vi "data insert core.vi"(8 "error in (no error)":errorcluster, 9 "column information":T1[](array[typedef]), 10 "data":variant[](array[variant]), 11 "table":string) -> (0 "error out":errorcluster)   [LabVIEW 2016, in "采配水.lvlib"]
uses:
  <vilib>/addons/database/Auxilliary.llb/DB Tools Column Info.ctl
  <vilib>/addons/database/Auxilliary.llb/DB Tools DataTypes.ctl
  <vilib>/Utility/sysdir.llb/System Directory Type.ctl
  <vilib>/addons/database/Auxilliary.llb/DB Tools Transaction.ctl
  <vilib>/addons/database/Auxilliary.llb/DB Tools Isolation Level.ctl
  <vilib>/addons/database/Auxilliary.llb/DB Tools Parameter Info.ctl
  <vilib>/addons/database/Auxilliary.llb/DB Tools Parameter Dir.ctl
  <vilib>/addons/database/Connection.llb/DB Tools Open Connec (String).vi
  <vilib>/addons/database/Connection.llb/Conn Transaction.vi
  <vilib>/addons/database/Connection.llb/Conn Execute.vi
  <vilib>/addons/database/Recordset.llb/Rec Destroy - Connection.vi
  <vilib>/addons/database/Command.llb/Cmd Set Parameter Value (C).vi
  <vilib>/addons/database/Auxilliary.llb/DB Tools Format Datetime String (Time Stamp).vi
  <vilib>/addons/database/Command.llb/Cmd Execute.vi
  <vilib>/addons/database/Recordset.llb/Rec Destroy - Command.vi
  <vilib>/addons/database/Command.llb/Cmd Delete.vi
  <vilib>/addons/database/NI_Database_API.lvlib
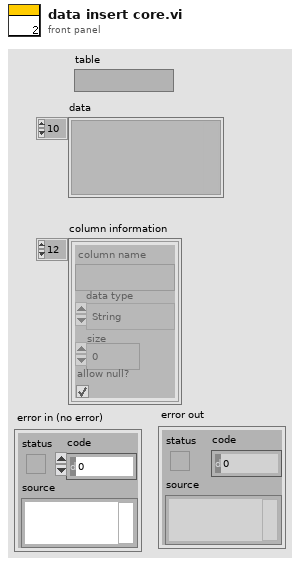
[diagram p1: front panel]
types:
  T1 = typedef "NI_Database_API.lvlib/DB Tools Column Info.ctl" = cluster{"column name":string, "data type":T2, "size":i32, "allow null?":bool}
  T2 = typedef "NI_Database_API.lvlib/DB Tools DataTypes.ctl" = enum16{"String", "Long (I32)", "Single (SGL)", "Double (DBL)", "Date/Time", "Binary"}
  T3 = typedef "NI_Database_API.lvlib/DB Tools Isolation Level.ctl" = enum16{"chaos", "read uncommitted", "read committed", "repeatable read", "serializable"}
  T4 = typedef "NI_Database_API.lvlib/DB Tools Transaction.ctl" = enum16{"begin", "commit", "rollback"}
  T5 = typedef "System Directory Type.ctl" = i32
  T6 = typedef "NI_Database_API.lvlib/Conn ObjectReference.ctl" = refnum<k1>
  T7 = typedef "NI_Database_API.lvlib/DB Tools Parameter Info.ctl" = cluster{"parameter name":string, "type":T2, "direction":T8, "value":variant}
  T8 = typedef "NI_Database_API.lvlib/DB Tools Parameter Dir.ctl" = enum32{"Input", "Output", "Input/Output", "Return Value"}
  T9 = typedef "NI_Database_API.lvlib/Rec ObjectReference.ctl" = refnum<k1>
  T10 = typedef "NI_Database_API.lvlib/Cmd ObjectReference.ctl" = refnum<k1>
  T11 = typedef "NI_Database_API.lvlib/Cmd-Rec Object Reference.ctl" = refnum<k1>
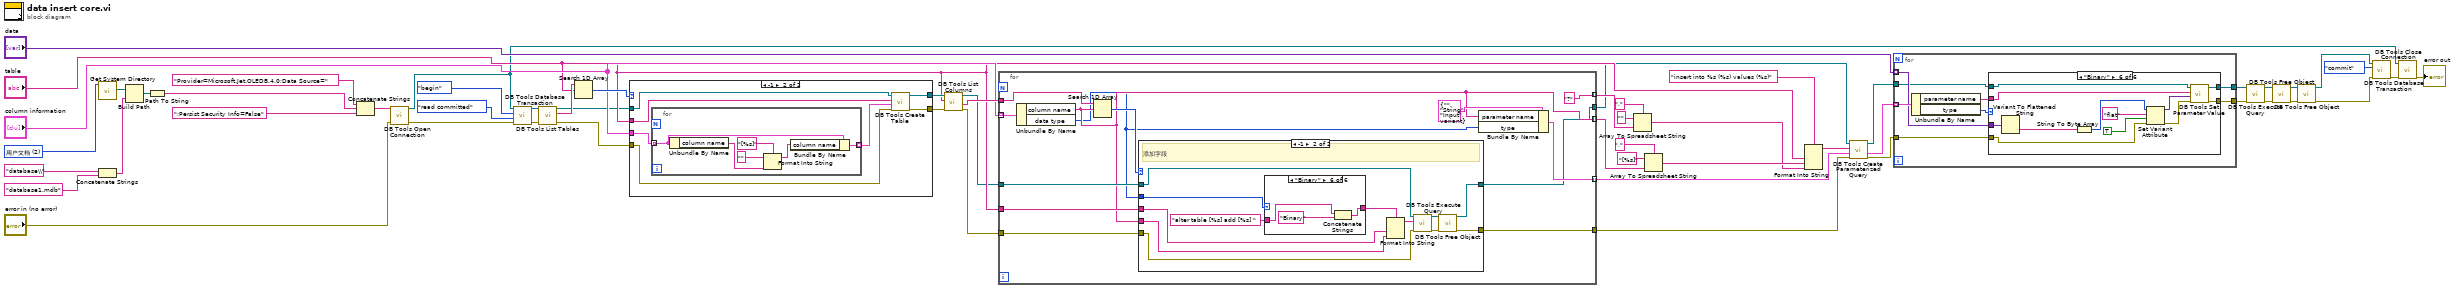
[diagram p0: block diagram]
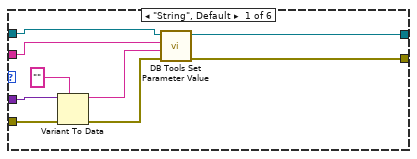
[diagram p2: hidden frame]
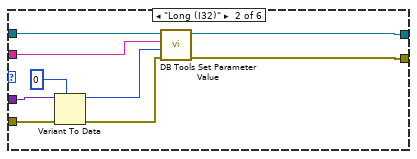
[diagram p3: hidden frame]
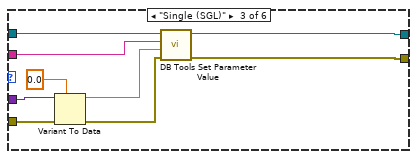
[diagram p4: hidden frame]
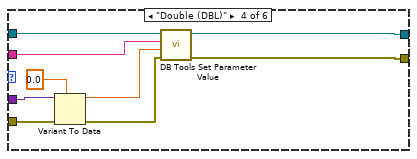
[diagram p5: hidden frame]
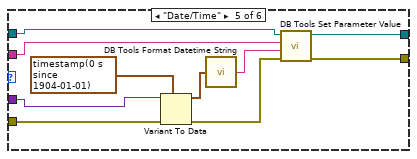
[diagram p6: hidden frame]
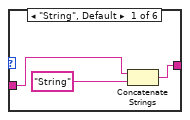
[diagram p8: hidden frame]
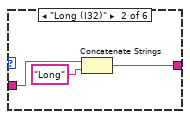
[diagram p9: hidden frame]
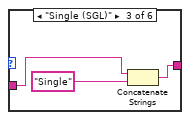
[diagram p10: hidden frame]
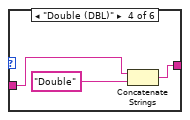
[diagram p11: hidden frame]
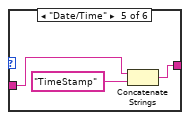
[diagram p12: hidden frame]
diagram:
  w56 = T5 2 items=["用户目录"=0, "用户桌面"=1, "用户文档"=2, "用户应用程序数据"=3, "用户设置"=4, "用户临时目录"=5, "公共文档"=6, "公共应用程序数据"=7, "公共设置"=8, "公共缓存"=13, "系统核心库"=9, "系统安装库"=10, "应用程序文件"=11, "启动盘根目录"=12] ("system directory type")
  n1 = call <vilib>:"Get System Directory.vi"("system directory type"=w56) -> ("system directory"=w54:path)  [unwired: 10 in]
  n2 = Concatenate Strings("database\\" ("condition"), "database1.mdb" ("database")) -> (w48:string)
  n3 = Build Path(base path=w54, name or relative path=w48) -> (appended path=w53:path)
  n4 = Path To String(path=w53) -> (string=w52:string)
  n5 = Concatenate Strings("Provider=Microsoft.Jet.OLEDB.4.0;Data Source=" ("condition"), w52, ";Persist Security Info=False" ("condition")) -> (w50:string)
  n6 = call-poly <vilib>:"DB Tools Open Connection.vi"("error in (no error)"="error in (no error)", "connection information"=w50) -> ("error out"=w9:errorcluster, "connection reference"=w1:T6)  [unwired: 6 in]
  n7 = call-poly <vilib>:"DB Tools Database Transaction.vi"("error in (no error)"=w9, "isolation level (chaos)"=DB_Tools_Isolation_Level."read committed", "operation (begin)"=DB_Tools_Transaction."begin", "connection reference"=w1) -> ("error out"=w8:errorcluster, "connection reference out"=w10:T6)  [unwired: 2 in]
  n8 = call <vilib>:"DB Tools List Tables.vi"("error in (no error)"=w8, "connection reference"=w10) -> ("error out"=w39:errorcluster, "tables"=w41:string[], "connection reference out"=w4:T6)  [unwired: 3 in]
  n9 = Search 1D Array(1D array=w41, element="table") -> (index of element=w40:i32)  [unwired: 1 in]
  n10 = case shown="-1" w40 {
    tunnel: w4 -> [w58 w65]
    tunnel: w39 -> [w57 w64]
    tunnel: "table" -> [_ w63]
    tunnel: "column information" -> [_ w60]
    tunnel: [w58 w62] -> w35
    tunnel: [w57 w61] -> w34
    frame 0, Default {
    }
    frame -1 {
      n11 = for {
        tunnel: w60 -> [w67] mode=indexing
        tunnel: [w66] -> w59 mode=indexing
        n12 = Unbundle By Name(w67) -> ("column name"=w71:string)
        n13 = Format Into String(format string="[%s]" ("格式字符串"), initial string="" ("初始字符串"), w71) -> (resulting string=w68:string)  [unwired: 1 in, 1 out]
        n14 = Bundle By Name(cluster=w67, "column name"=w68) -> (w66:T1)
      }
      n15 = call <vilib>:"DB Tools Create Table.vi"("error in (no error)"=w64, "column information"=w59, "table"=w63, "connection reference"=w65) -> ("error out"=w61:errorcluster, "connection reference out"=w62:T6)  [unwired: 4 in]
    }
  }
  n16 = call <vilib>:"DB Tools List Columns.vi"("error in (no error)"=w34, "table"="table", "connection reference"=w35) -> ("error out"=w37:errorcluster, "columns"=w38:string[], "connection reference out"=w6:T6)  [unwired: 1 in, 1 out]
  n17 = for {
    tunnel: w6 -> [w82]
    tunnel: w38 -> [w84]
    tunnel: w37 -> [w81]
    tunnel: [w80] -> w33
    tunnel: "table" -> [w79]
    tunnel: "column information" -> [w78] mode=indexing
    tunnel: [w76] -> w32 mode=indexing
    tunnel: [w75] -> w25 mode=indexing
    tunnel: ["?"] -> w23 mode=indexing
    tunnel: [w72] -> w3
    n18 = Unbundle By Name(w78) -> ("column name"=w75:string, "data type"=w73:T2)
    n19 = Search 1D Array(1D array=w84, element=w75) -> (index of element=w83:i32)  [unwired: 1 in]
    n20 = case shown="-1" w83 {
      tunnel: [w86 w95] -> w80
      tunnel: w82 -> [w85 w94]
      tunnel: w75 -> [_ w93]
      tunnel: w81 -> [w86 w92]
      tunnel: w79 -> [_ w91]
      tunnel: w73 -> [_ w89]
      tunnel: [w85 w87] -> w72
      frame 0, Default {
      }
      frame -1 {
        # "添加字段"
        n21 = case shown="\"Binary\"" w89 {
          tunnel: "alter table [%s] add [%s] " -> [w101 w104 w107 w110 w113 w116]
          tunnel: [w100 w103 w106 w109 w112 w115] -> w88
          frame "String", Default {
            n22 = Concatenate Strings(w101, "String" ("字符串")) -> (w100:string)
          }
          frame "Long (I32)" {
            n23 = Concatenate Strings(w104, "Long" ("字符串")) -> (w103:string)
          }
          frame "Single (SGL)" {
            n24 = Concatenate Strings(w107, "Single" ("字符串")) -> (w106:string)
          }
          frame "Double (DBL)" {
            n25 = Concatenate Strings(w110, "Double" ("字符串")) -> (w109:string)
          }
          frame "Date/Time" {
            n26 = Concatenate Strings(w113, "TimeStamp" ("字符串")) -> (w112:string)
          }
          frame "Binary" {
            n27 = Concatenate Strings(w116, "Binary" ("字符串")) -> (w115:string)
          }
        }
        n28 = Format Into String(format string=w88, w91, w93) -> (resulting string=w96:string)  [unwired: 2 in, 1 out]
        n29 = call-poly <vilib>:"DB Tools Execute Query.vi"("error in (no error)"=w92, "SQL query"=w96, "connection reference"=w94) -> ("error out"=w97:errorcluster, "recordset reference"=w98:T9)  [unwired: 5 in]
        n30 = call-poly <vilib>:"DB Tools Free Object.vi"("error in (no error)"=w97, "recordset reference"=w98) -> ("error out"=w95:errorcluster, "connection reference"=w87:T6)  [unwired: 8 in]
      }
    }
    n31 = Bundle By Name(cluster=T7 {"parameter name"="", "type"=enum."String", "direction"=enum."Input", "value"=variant} ("parameter information"), "parameter name"=w75, "type"=w73) -> (w76:T7)
  }
  n32 = Array To Spreadsheet String(delimiter (Tab)="," ("分隔符(Tab)"), array=w23, 3:"" ("格式字符串")) -> (spreadsheet string=w22:string)
  n33 = Array To Spreadsheet String(delimiter (Tab)="," ("分隔符(Tab)"), array=w25, 3:"[%s]" ("格式字符串")) -> (spreadsheet string=w24:string)
  n34 = Format Into String(format string="insert into %s (%s) values (%s)" ("格式字符串"), "table", w24, w22) -> (resulting string=w21:string)  [unwired: 2 in, 1 out]
  n35 = call <vilib>:"DB Tools Create Parameterized Query.vi"("error in (no error)"=w33, "parameters"=w32, "SQL query"=w21, "connection reference"=w3) -> ("error out"=w20:errorcluster, "parameters out"=w19:T7[], "command reference"=w5:T10)  [unwired: 3 in]
  n36 = for {
    tunnel: w5 -> [w121]
    tunnel: w20 -> [w119]
    tunnel: w19 -> [w124] mode=indexing
    tunnel: "data" -> [w122] mode=indexing
    tunnel: [w118] -> w2
    tunnel: [w117] -> w18
    n37 = Unbundle By Name(w124) -> ("parameter name"=w120:string, "type"=w123:T2)
    n38 = case shown="\"Binary\"" w123 {
      tunnel: w122 -> [w128 w136 w143 w153 w170 w174]
      tunnel: w121 -> [w131 w140 w147 w157 w168 w182]
      tunnel: w120 -> [w130 w139 w146 w152 w167 w181]
      tunnel: w119 -> [w125 w134 w144 w154 w165 w173]
      tunnel: [w127 w138 w148 w156 w164 w180] -> w118
      tunnel: [w126 w137 w145 w155 w163 w179] -> w117
      frame "String", Default {
        n39 = Variant To Data(error in=w125, type="", Variant=w128) -> (data=w129:string, error out=w133:errorcluster)
        n40 = call-poly <vilib>:"DB Tools Set Parameter Value.vi"("error in (no error)"=w133, "value"=w129, "parameter index"=w130, "command reference"=w131) -> ("error out"=w126:errorcluster, "command reference out"=w127:T10)  [unwired: 4 in]
      }
      frame "Long (I32)" {
        n41 = Variant To Data(error in=w134, type=0, Variant=w136) -> (data=w141:i32, error out=w142:errorcluster)
        n42 = call-poly <vilib>:"DB Tools Set Parameter Value.vi"("error in (no error)"=w142, "value"=w141, "parameter index"=w139, "command reference"=w140) -> ("error out"=w137:errorcluster, "command reference out"=w138:T10)  [unwired: 4 in]
      }
      frame "Single (SGL)" {
        n43 = Variant To Data(error in=w144, type=sgl 0.0, Variant=w143) -> (data=w150:sgl, error out=w151:errorcluster)
        n44 = call-poly <vilib>:"DB Tools Set Parameter Value.vi"("error in (no error)"=w151, "value"=w150, "parameter index"=w146, "command reference"=w147) -> ("error out"=w145:errorcluster, "command reference out"=w148:T10)  [unwired: 4 in]
      }
      frame "Double (DBL)" {
        n45 = Variant To Data(error in=w154, type=0.0, Variant=w153) -> (data=w159:dbl, error out=w160:errorcluster)
        n46 = call-poly <vilib>:"DB Tools Set Parameter Value.vi"("error in (no error)"=w160, "value"=w159, "parameter index"=w152, "command reference"=w157) -> ("error out"=w155:errorcluster, "command reference out"=w156:T10)  [unwired: 4 in]
      }
      frame "Date/Time" {
        n47 = Variant To Data(error in=w165, type=timestamp(0 s since 1904-01-01) ("时间标识"), Variant=w170) -> (data=w162:timestamp, error out=w166:errorcluster)
        n48 = call-poly <vilib>:"DB Tools Format Datetime String.vi"("time stamp"=w162) -> ("date/time string"=w161:string)
        n49 = call-poly <vilib>:"DB Tools Set Parameter Value.vi"("error in (no error)"=w166, "value"=w161, "parameter index"=w167, "command reference"=w168) -> ("error out"=w163:errorcluster, "command reference out"=w164:T10)  [unwired: 4 in]
      }
      frame "Binary" {
        n50 = Variant To Flattened String(Variant=w174) -> (data string=w175:string)  [unwired: 1 out]
        n51 = String To Byte Array(string=w175) -> (unsigned byte array=w178:u8[])
        n52 = Set Variant Attribute(Variant=w178, name="flat", value=TRUE, error in=w173) -> (Variant out=w171:variant, error out=w172:errorcluster)  [unwired: 1 out]
        n53 = call-poly <vilib>:"DB Tools Set Parameter Value.vi"("error in (no error)"=w172, "value"=w171, "parameter index"=w181, "command reference"=w182) -> ("error out"=w179:errorcluster, "command reference out"=w180:T10)  [unwired: 4 in]
      }
    }
  }
  n54 = call-poly <vilib>:"DB Tools Execute Query.vi"("error in (no error)"=w18, "command reference"=w2) -> ("error out"=w16:errorcluster, "command-recordset reference"=w17:T11)  [unwired: 6 in]
  n55 = call-poly <vilib>:"DB Tools Free Object.vi"("error in (no error)"=w16, "command-recordset reference"=w17) -> ("error out"=w14:errorcluster, "command reference"=w15:T10)  [unwired: 8 in]
  n56 = call-poly <vilib>:"DB Tools Free Object.vi"("error in (no error)"=w14, "command reference"=w15) -> ("error out"=w11:errorcluster, "connection reference"=w12:T6)  [unwired: 8 in]
  n57 = call-poly <vilib>:"DB Tools Database Transaction.vi"("error in (no error)"=w11, "operation (begin)"=DB_Tools_Transaction."commit", "connection reference"=w12) -> ("error out"=w13:errorcluster)  [unwired: 3 in, 1 out]
  n58 = call <vilib>:"DB Tools Close Connection.vi"("error in (no error)"=w13, "connection reference"=w1) -> ("error out"=→"error out":errorcluster)  [unwired: 5 in]
